vi "Cloud <-> OpenMV.vi"() -> ()   [LabVIEW 2019]
uses:
  <userlib>/MicroPython/VIs/uPythonX/uPythonX.xctl
panel:
  in  "OM_urequests":T1(xcontrol)={"Port"="OpenMV - ASRL12::INSTR", "All Code"="import usocket\n\ndebug = 0\n\nimport uio\nclass SocketWrap(uio.IOBase):\n    def __init__(self, s):\n        self.s = s\n    def connect(self, x):\n        print('connect', x)\n        return self.s.connect(x)\n    def close(self):\n        print('close')\n        return self.s.close()\n    def write(self, x):\n        import binascii\n        print('write', len(x), binascii.hexlify(x))\n        return self.s.write(x)\n    def readinto(self, x):\n        import binascii\n        ret = self.s.readinto(x)\n        print('readinto', len(x), ret, binascii.hexlify(x))\n        return ret\n    def ioctl(self, x, y):\n        print('ioctl', x, y)\n        if x == 4: # close\n            self.s.close()\n            return 0\n        else:\n            return self.s.ioctl(x, y)\n\nclass Response:\n\n    def __init__(self, f):\n        self.raw = f\n        self.encoding = \"utf-8\"\n        self._cached = None\n\n    def close(self):\n        if self.raw:\n            self.raw.close()\n            self.raw = None\n        self._cached = None\n\n    @property\n    def content(self):\n        if self._cached is None:\n            try:\n                self._cached = self.raw.read()\n            finally:\n                self.raw.close()\n                self.raw = None\n        return self._cached\n\n    @property\n    def text(self):\n        return str(self.content, self.encoding)\n\n    def json(self):\n        import ujson\n        return ujson.loads(self.content)\n\n\ndef request(method, url, data=None, json=None, headers={}, stream=None):\n    try:\n        proto, dummy, host, path = url.split(\"/\", 3)\n    except ValueError:\n        proto, dummy, host = url.split(\"/\", 2)\n        path = \"\"\n    if proto == \"http:\":\n        port = 80\n    elif proto == \"https:\":\n        import ussl\n        port = 443\n    else:\n        raise ValueError(\"Unsupported protocol: \" + proto)\n\n    if \":\" in host:\n        host, port = host.split(\":\", 1)\n        port = int(port)\n    #print(host,port)\n    ai = usocket.getaddrinfo(host,port)[0][4]\n\n    s = usocket.socket(usocket.AF_INET, usocket.SOCK_STREAM)\n    if debug:\n        s = SocketWrap(s)\n    try:\n        s.connect(ai)\n        if proto == \"https:\":\n            if debug:\n                print('wrap')\n            s = ussl.wrap_socket(s, server_hostname=host)\n            if debug:\n                print('wrap done')\n        s.write(b\"%s /%s HTTP/1.0\\r\\n\" % (method, path))\n        if not \"Host\" in headers:\n            s.write(b\"Host: %s\\r\\n\" % host)\n        # Iterate over keys to avoid tuple alloc\n        for k in headers:\n            s.write(k)\n            s.write(b\": \")\n            s.write(headers[k])\n            s.write(b\"\\r\\n\")\n        if json is not None:\n            assert data is None\n            import ujson\n            data = ujson.dumps(json)\n            s.write(b\"Content-Type: application/json\\r\\n\")\n        if data:\n            s.write(b\"Content-Length: %d\\r\\n\" % len(data))\n        s.write(b\"\\r\\n\")\n        if data:\n            s.write(data)\n\n        l = s.readline()\n        #print(l)\n        l = l.split(None, 2)\n        status = int(l[1])\n        reason = \"\"\n        if len(l) > 2:\n            reason = l[2].rstrip()\n        while True:\n            l = s.readline()\n            if not l or l == b\"\\r\\n\":\n                break\n            #print(l)\n            if l.startswith(b\"Transfer-Encoding:\"):\n                if b\"chunked\" in l:\n                    raise ValueError(\"Unsupported \" + l)\n            elif l.startswith(b\"Location:\") and not 200 <= status <= 299:\n                raise NotImplementedError(\"Redirects not yet supported\")\n    except OSError:\n        s.close()\n        raise\n    if debug:\n        print('headers done')\n\n    resp = Response(s)\n    resp.status_code = status\n    resp.reason = reason\n    return resp\n\n\ndef head(url, **kw):\n    return request(\"HEAD\", url, **kw)\n\ndef get(url, **kw):\n    return request(\"GET\", url, **kw)\n\ndef post(url, **kw):\n    return request(\"POST\", url, **kw)\n\ndef put(url, **kw):\n    return request(\"PUT\", url, **kw)\n\ndef patch(url, **kw):\n    return request(\"PATCH\", url, **kw)\n\ndef delete(url, **kw):\n    return request(\"DELETE\", url, **kw)\n\n'''if debug:\n    import net\n    net.wlan_connect()\n    get('https://192.168.1.88:8443/').text\n'''\n"}
  in  "main":T1(xcontrol)={"Port"="OpenMV - ASRL12::INSTR", "All Code"="import machine, network, ubinascii, ujson,  utime, gc\nimport OM_urequests as urequests\nimport passwords\n\nWiFi = network.WINC()\nWiFi.isconnected()\n\ndef connect():\n     while not WiFi.isconnected():\n          print (\"Connecting ..\")\n          WiFi.connect(passwords.wifi['username'],passwords.wifi['password'],security=WiFi.WPA_PSK)\n          print(WiFi.ifconfig())\n          i=0\n          while i < 25 and not WiFi.isconnected():\n               utime.sleep_ms(200)\n               i=i+1\n          print (\"WiFi: \",WiFi.isconnected())\n          if i == 25:\n               utime.sleep(1)\n     return WiFi.isconnected()\n\ndef connect2():\n     print (\"Connecting ..\")\n     WiFi.connect(passwords.wifi['username'],passwords.wifi['password'],security=WiFi.WPA_PSK)\n     print(WiFi.ifconfig())\n     i=0\n     while i < 25 and not WiFi.isconnected():\n          utime.sleep_ms(200)\n          i=i+1\n     print (\"WiFi: \",WiFi.isconnected())\n     if i == 25:\n          utime.sleep(1)\n     return WiFi.isconnected()\n\ndef SL_setup():\n     urlBase = \"https://api.systemlinkcloud.com/nitag/v2/tags/\"\n     Key = passwords.Keys['SystemLink']\n     headers = {\"Accept\":\"application/json\",\"x-ni-api-key\":Key}\n     return urlBase, headers\n\ndef Get_SL(Tag):\n     urlBase, headers = SL_setup()\n     urlValue = urlBase + Tag + \"/values/current\"\n     try:\n          value = urequests.get(urlValue,headers=headers).text\n          #print(value)\n          data = ujson.loads(value)\n          result = data.get(\"value\").get(\"value\")\n     except Exception as e:\n          print(e)\n          result = e\n     return result\n\ndef Put_SL(Tag, Type, Value):\n     urlBase, headers = SL_setup()\n     urlTag = urlBase + Tag\n     urlValue = urlBase + Tag + \"/values/current\"\n     propName={\"type\":Type,\"path\":Tag}\n     propValue = {\"value\":{\"type\":Type,\"value\":Value}}\n     try:\n          callTag = urequests.put(urlTag,headers=headers,json=propName).text\n     except Exception as e:\n          print(e)\n     try:\n          callValue = urequests.put(urlValue,headers=headers,json=propValue).text\n     except Exception as e:\n          print(e)\n          callValue = ''\n     return callValue\n\nconnect2()\ni = 0\nwhile 1:\n     i += 1\n     Get_SL('fred_Num')\n     Put_SL('fred_Num','INT',str(i))\n     Get_SL('fred_Num')\n     utime.sleep(1)\n     gc.collect()\n\n'''\nimport usocket\nTag = 'HP_Geo_T0'\r\nurlBase, headers = SL_setup()\r\nurlValue = urlBase + Tag + \"/values/current\"\nproto, dummy, host, path = urlValue.split(\"/\", 3)\nif proto == \"http:\":\n   port = 80\nif proto == \"https:\":\n   import ussl\n   port = 443\nWiFi = network.WINC()\nWiFi.connect('HighPeaks','s0meth1ng',security=WiFi.WPA_PSK)\nWiFi.ifconfig()\nai = usocket.getaddrinfo(host,port)[0][4]\ns = usocket.socket(usocket.AF_INET, usocket.SOCK_STREAM)\ns.connect(ai)\ns = ussl.wrap_socket(s, server_hostname=host)\ns.write(b\"%s /%s HTTP/1.0\\r\\n\" % ('GET', path))\n\r\nurequests.get(urlValue,headers=headers).text\n\nWiFi.ifconfig()\nusocket.getaddrinfo('api.systemlinkcloud.com',443)[0][4]\n\n'''"}
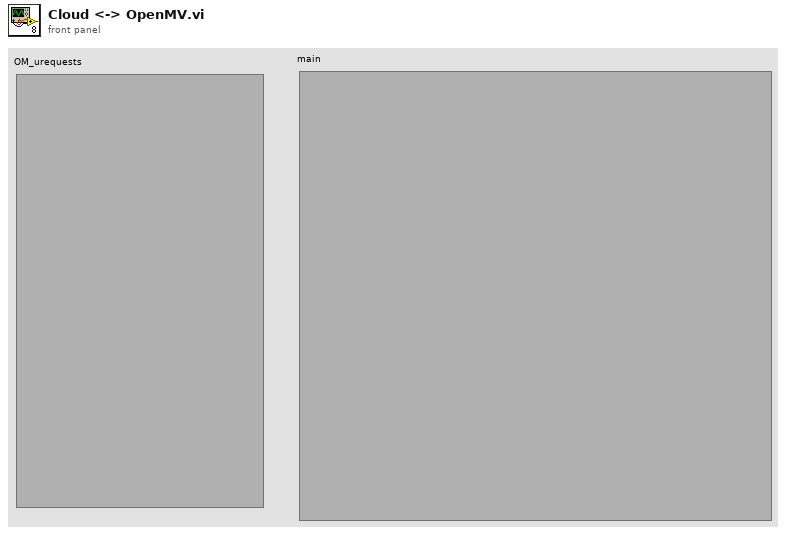
[diagram p1: front panel]
types:
  T1 = cluster{"Port":refnum<visa-resource-name>, "All Code":string}
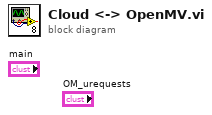
[diagram p0: block diagram]
diagram:
